vi "Untitled 5 (SubVI).vi"(10 "Variant":variant, 11 "Refnums":refnum<file>[](array[refnum])) -> (3 "Refnums 2":refnum<file>[](array[refnum]))   [LabVIEW 2015]
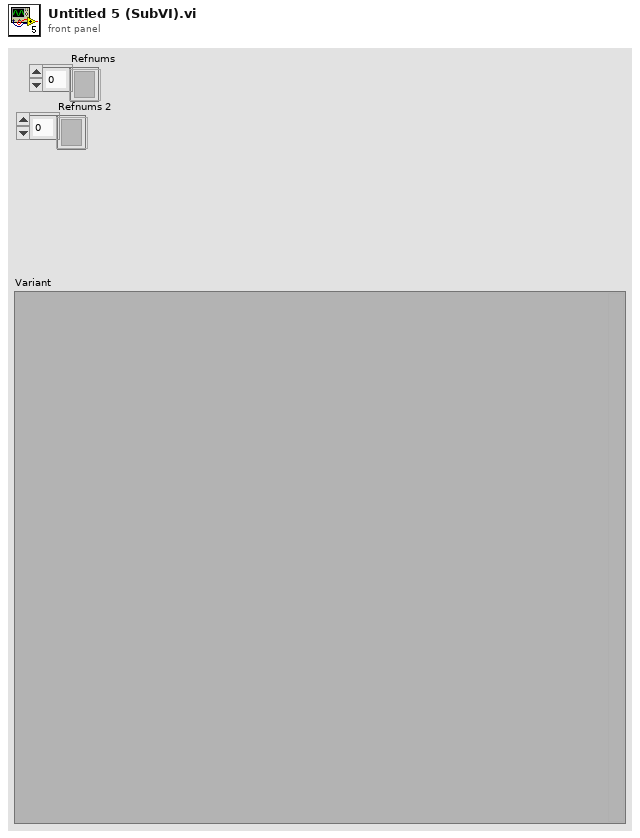
[diagram p1: front panel]
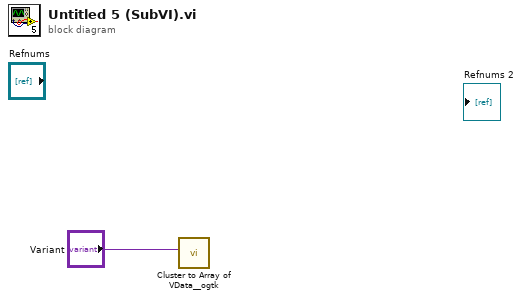
[diagram p0: block diagram]
diagram:
  n1 = call <userlib>:"Cluster to Array of VData__ogtk.vi"("Cluster"="Variant") -> ()  [unwired: 9 in, 2 out]
